vi "Symphony Acquire Image Clean.vi"(5 "Acquire":refnum<vi>, 7 "Running":refnum<vi>, 8 "error in":errorcluster caption="entrée d'erreur (pas d'erreur)", 10 "ShutterOpen":bool, 11 "JYCCDLib.IJYCCDReqd":refnum<k7>) -> (0 "Acq Time(ms)":u32, 3 "Raw Data":i32[][][](array[numeric]))   [LabVIEW 2010]
panel:
  out "AcquisitionBusy":bool
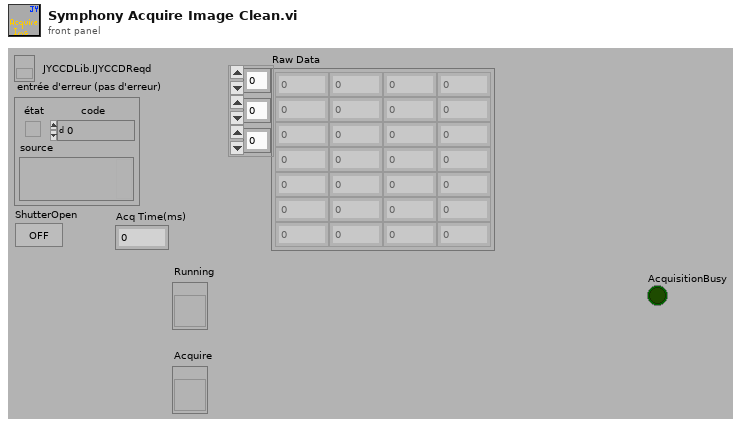
[diagram p1: front panel]
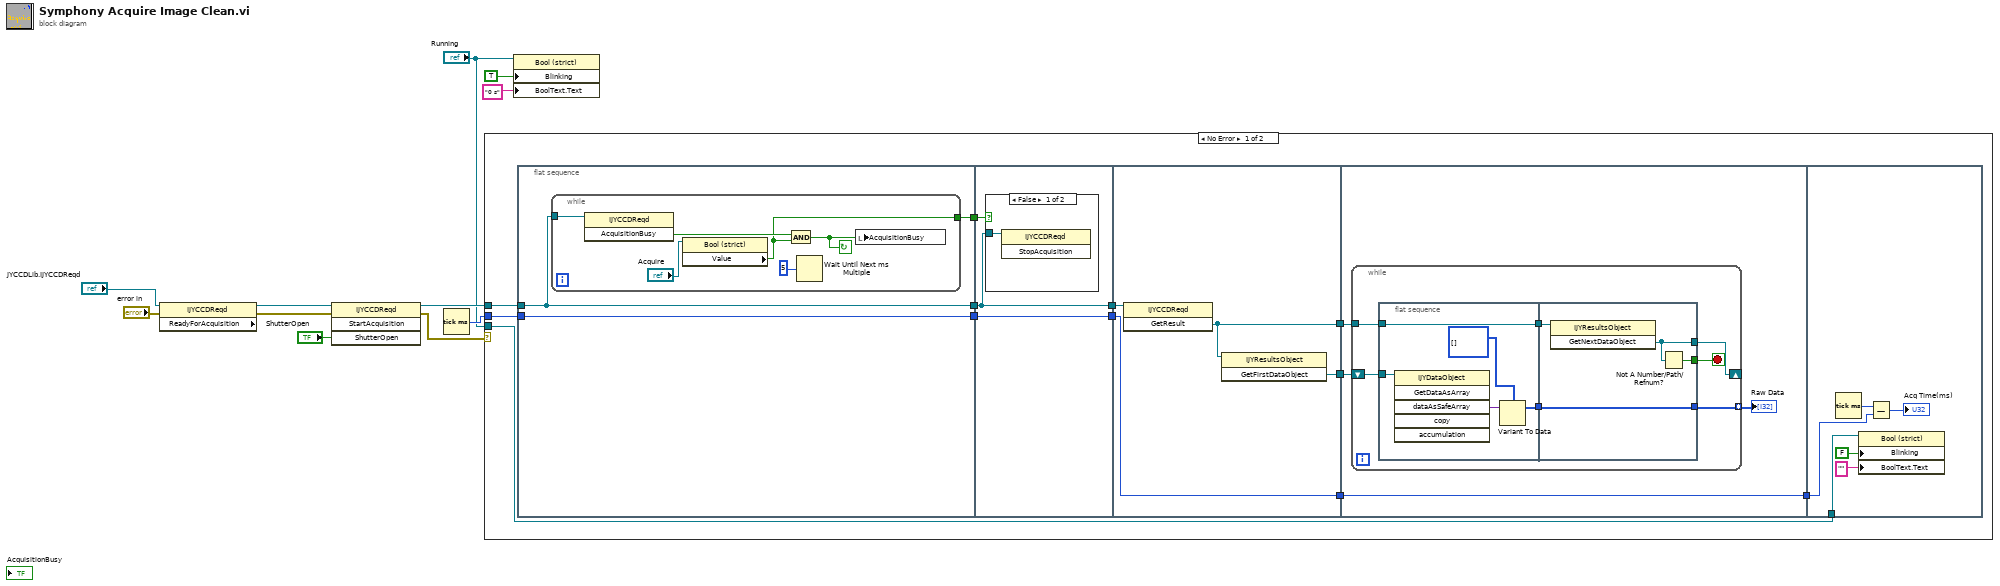
[diagram p0: block diagram]
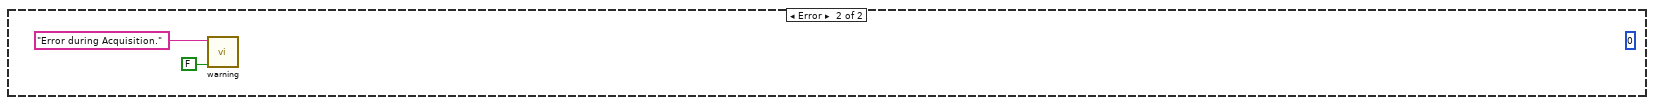
[diagram p3: hidden frame]
diagram:
  n1 = property class="IJYCCDReqd" props=["ReadyForAcquisition"](reference="JYCCDLib.IJYCCDReqd", error in="error in") -> (reference out=w6:refnum<k7>, error out=w5:errorcluster)  [unwired: 1 out]
  n2 = invoke class="IJYCCDReqd" method="StartAcquisition"(reference=w6, error in=w5, "ShutterOpen"="ShutterOpen") -> (reference out=w11:refnum<k7>, error out=w9:errorcluster)  [unwired: 1 in, 2 out]
  n3 = Tick Count (ms)() -> (millisecond timer value=w10:u32)
  n4 = case shown="No Error" w9 {
    tunnel: w11 -> [w23 _]
    tunnel: w10 -> [w22 _]
    tunnel: "Running" -> [w12 _]
    frame No Error {
      n5 = flat-sequence {
        tunnel: w23 -> [w26]
        tunnel: [w26] -> w17
        tunnel: w22 -> [w25]
        tunnel: [w25] -> w15
        tunnel: [w24] -> w13
        tunnel: w17 -> [w33]
        tunnel: [w33] -> w16
        tunnel: w15 -> [w35]
        tunnel: [w35] -> w14
        tunnel: w13 -> [w34]
        tunnel: w16 -> [w40]
        tunnel: w14 -> [w37]
        tunnel: [w37] -> w21
        tunnel: [w39] -> w20
        tunnel: [w38] -> w19
        tunnel: w21 -> [w41]
        tunnel: [w41] -> w18
        tunnel: w20 -> [w44]
        tunnel: w19 -> [w43]
        tunnel: w18 -> [w65]
        tunnel: w12 -> [w61]
        frame #0 {
          n6 = while {
            tunnel: w26 -> [w32]
            tunnel: [w27] -> w24
            stop <- w28 continue-if-true
            n7 = invoke class="IJYCCDReqd" method="AcquisitionBusy"(reference=w32) -> ("AcquisitionBusy"=w29:bool)  [unwired: 2 in, 2 out]
            n8 = property class="Bool (strict)"(reference="Acquire") -> ("Value"=w27:bool)  [unwired: 1 in, 2 out]
            n9 = And(x=w29, y=w27) -> (x .and. y?=w28:bool)
            n10 = Wait Until Next ms Multiple(millisecond multiple=u32 5 ("n millisecondes")) -> ()  [unwired: 1 out]
            n11 = local write "AcquisitionBusy"(w28) -> ()
          }
        }
        frame #1 {
          n12 = case shown="False" w34 {
            tunnel: w33 -> [w36 _]
            frame False {
              n13 = invoke class="IJYCCDReqd" method="StopAcquisition"(reference=w36) -> ()  [unwired: 2 in, 3 out]
            }
            frame True {
            }
          }
        }
        frame #2 {
          n14 = invoke class="IJYCCDReqd" method="GetResult"(reference=w40) -> ("GetResult"=w38:refnum<k7>)  [unwired: 2 in, 2 out]
          n15 = invoke class="IJYResultsObject" method="GetFirstDataObject"(reference=w38) -> ("GetFirstDataObject"=w39:refnum<k7>)  [unwired: 2 in, 2 out]
        }
        frame #3 {
          n16 = while {
            tunnel: [w48] -> w42 mode=indexing
            tunnel: w43 -> [w50]
            shift-left: w44 -> [w51]
            shift-right: [w49] -> _
            stop <- w47 stop-if-true
            n17 = flat-sequence {
              tunnel: w51 -> [w54]
              tunnel: w50 -> [w52]
              tunnel: [w52] -> w46
              tunnel: [w53] -> w45
              tunnel: w46 -> [w60]
              tunnel: [w59] -> w49
              tunnel: [w57] -> w48
              tunnel: w45 -> [w57]
              tunnel: [w58] -> w47
              frame #0 {
                n18 = invoke class="IJYDataObject" method="GetDataAsArray"(reference=w54) -> ("dataAsSafeArray"=w55:variant)  [unwired: 5 in, 5 out]
                n19 = Variant To Data(Variant=w55, type=i32[][] []) -> (data=w53:i32[][])  [unwired: 1 in, 1 out]
              }
              frame #1 {
                n20 = invoke class="IJYResultsObject" method="GetNextDataObject"(reference=w60) -> ("GetNextDataObject"=w59:refnum<k7>)  [unwired: 2 in, 2 out]
                n21 = Not A Number/Path/Refnum?(number/path/refnum=w59) -> (NaN/Path/Refnum?=w58:bool)
              }
            }
          }
          "Raw Data" <- w42
        }
        frame #4 {
          n22 = Tick Count (ms)() -> (millisecond timer value=w66:u32)
          n23 = property class="Bool (strict)"(reference=w61, "Blinking"=FALSE ("Blinkend"), "BoolText.Text"="" ("Boolean Text.Text")) -> ()  [unwired: 1 in, 2 out]
          n24 = Subtract(x=w66, y=w65) -> (x-y=→"Acq Time(ms)":u32)
        }
      }
    }
    frame Error {
      (unwired) u32 0 ("millisecond timer value")
      n25 = call "warning.vi"("with cancel ?"=FALSE, "Text"="Error during Acquisition.") -> ()  [unwired: 2 in, 1 out]
    }
  }
  n26 = property class="Bool (strict)"(reference="Running", "Blinking"=TRUE ("Blinkend"), "BoolText.Text"="0 s" ("Boolean Text.Text")) -> ()  [unwired: 1 in, 2 out]
